vi "Create Fill.vi"(8 "error in":errorcluster, 10 "PatternType":string, 11 "SpreadsheetDoc in":refnum<k24>) -> (0 "error out":errorcluster, 3 "SpreadsheetDoc out":refnum<k24>)   [LabVIEW 2021, in "Open Xml.lvlib"]
uses:
  Open Xml.lvlib
  D:/git/Open-Xml-LabVIEW/dll/DocumentFormat.OpenXml.dll
  dll/DocumentFormat.OpenXml.dll
  D:/git/Open-Xml-LabVIEW/dll/DocumentFormat.OpenXml.Framework.dll
  dll/DocumentFormat.OpenXml.Framework.dll
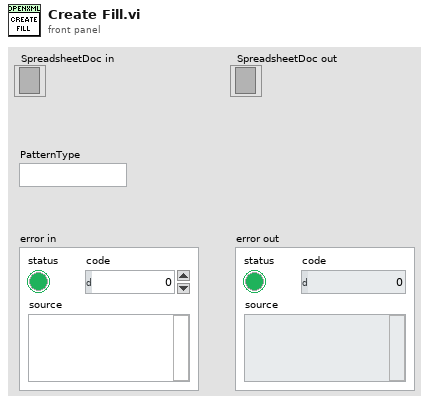
[diagram p1: front panel]
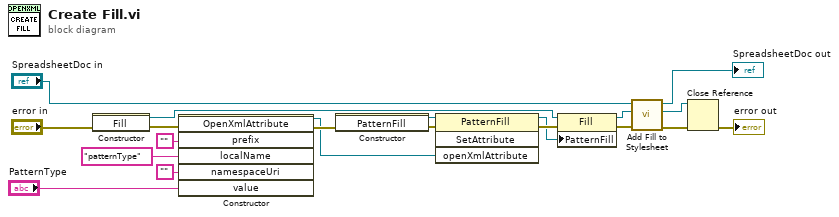
[diagram p0: block diagram]
diagram:
  n1 = constructor class="Fill"(error in="error in") -> (reference out=w6:refnum<k24>, error out=w17:errorcluster)  [unwired: 2 in, 1 out]
  n2 = constructor class="OpenXmlAttribute"(error in=w17, "prefix"="", "localName"="patternType", "namespaceUri"="", "value"="PatternType") -> (reference out=w12:refnum<k24>, error out=w18:errorcluster)  [unwired: 2 in, 5 out]
  n3 = constructor class="PatternFill"(error in=w18) -> (reference out=w8:refnum<k24>, error out=w10:errorcluster)  [unwired: 2 in, 1 out]
  n4 = invoke class="PatternFill" method="SetAttribute"(reference=w8, error in=w10, "openXmlAttribute"=w12) -> (reference out=w9:refnum<k24>, error out=w11:errorcluster)  [unwired: 1 in, 2 out]
  n5 = property class="Fill"(reference=w6, error in=w11, "PatternFill"=w9) -> (reference out=w7:refnum<k24>, error out=w5:errorcluster)
  n6 = call "Add Fill to Stylesheet.vi"("error in"=w5, "Fill in"=w7, "SpreadsheetDoc in"="SpreadsheetDoc in") -> ("error out"=w3:errorcluster, "Fill out"=w4:refnum<k24>, "SpreadsheetDoc out"=→"SpreadsheetDoc out":refnum<k24>)  [unwired: 5 in, 1 out]
  n7 = Close Reference(reference=w4, error in (no error)=w3) -> (error out=→"error out":errorcluster)
